vi "split data.vi"(6 "Slide":cluster{dbl, dbl}(slide)={0.0, 1.2121212121212122} scale=-0.00049998..0.0004999999999996373, 7 "dt":dbl, 8 "t0":dbl, 9 "Y(input)":dbl[](array[numeric]), 10 "T(input)":dbl[](array[numeric])) -> (0 "max value":dbl, 1 "min value":dbl, 2 "Y(output)":dbl[](array[numeric]), 3 "T(output)":dbl[](array[numeric]))   [LabVIEW 2014]
panel:
  out "XY Graph":cluster{"T(input)":dbl[], "Y(input) ":dbl[]}(graph)
  out "min index(es)":i32
  out "max index(es)":i32
  out "max":dbl
  out "min":dbl
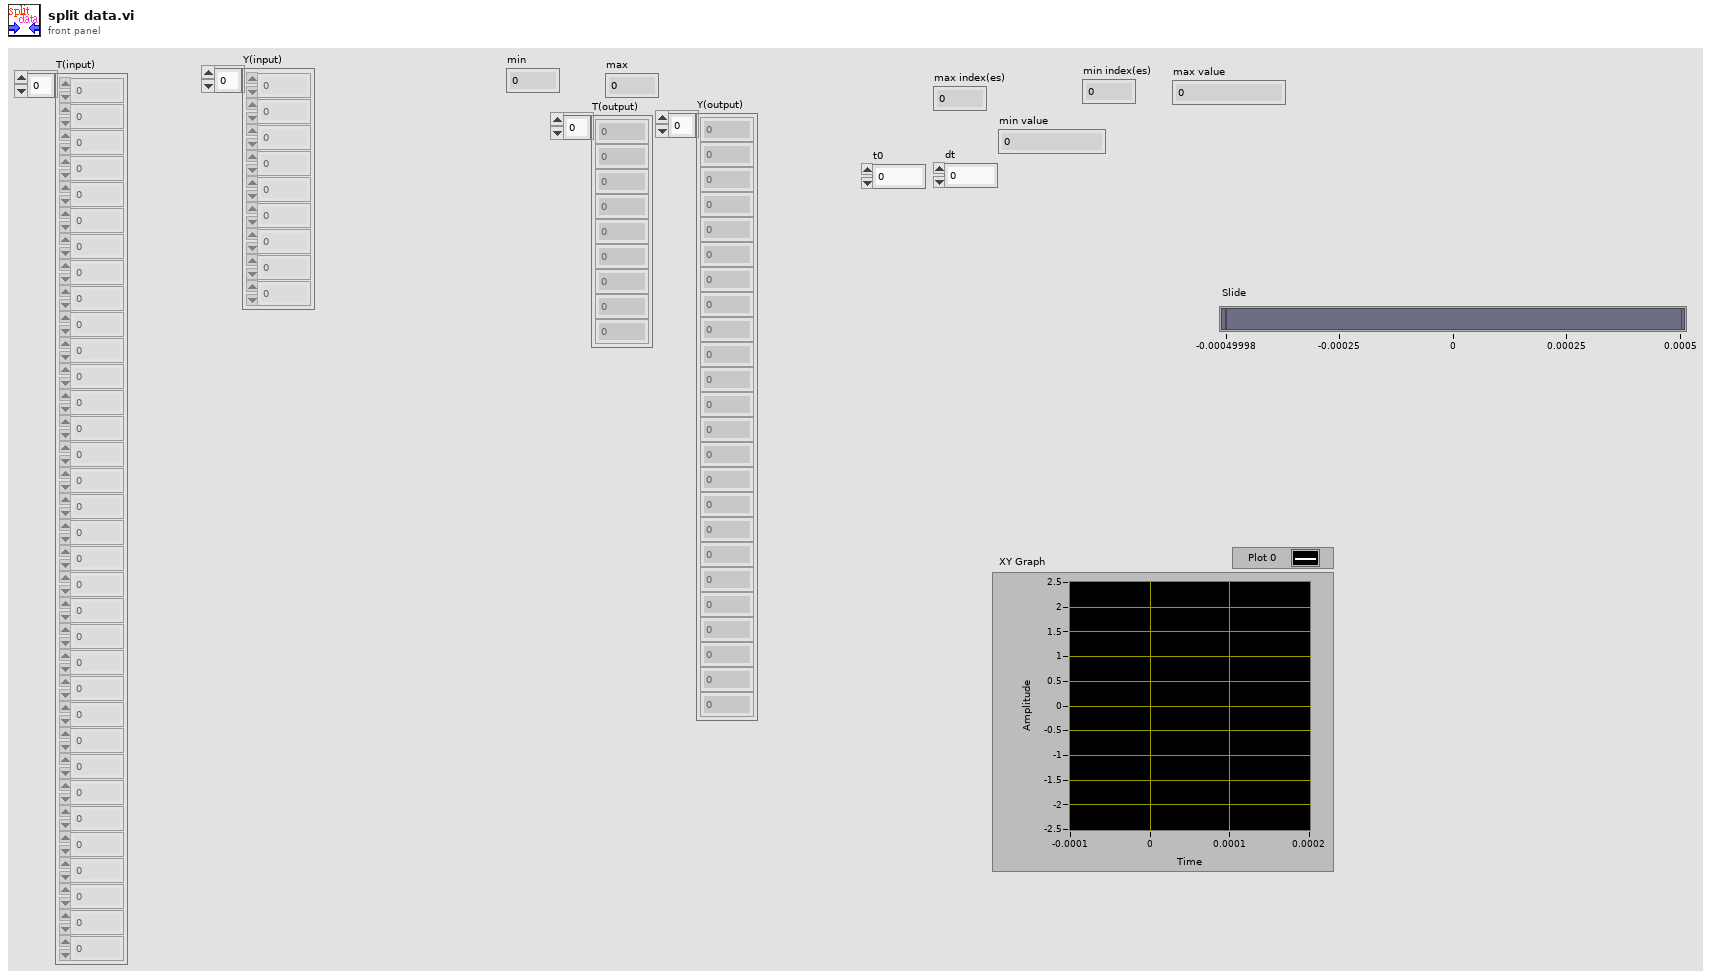
[diagram p1: front panel]
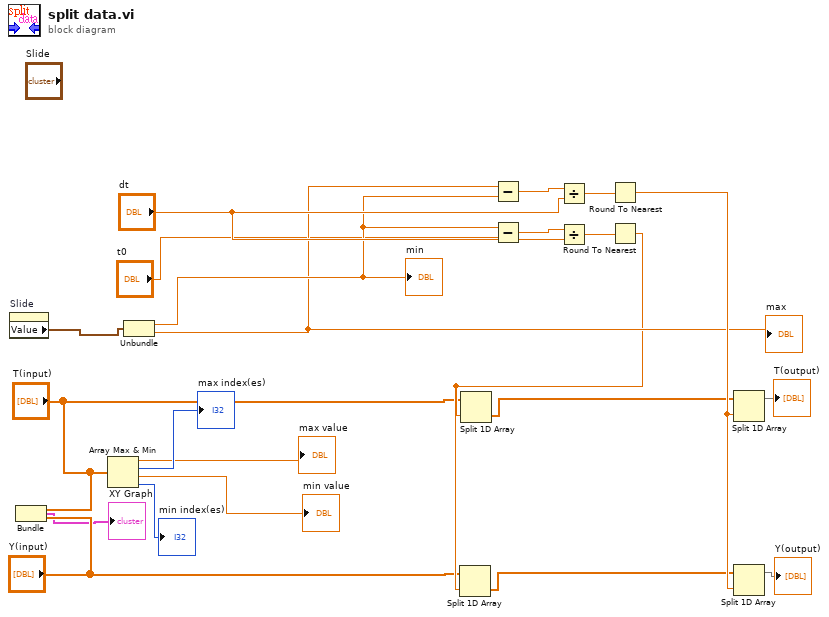
[diagram p0: block diagram]
diagram:
  n1 = property on="Slide" class="Slide (strict)"() -> ("Value"=w6:cluster{dbl, dbl})  [unwired: 2 in, 2 out]
  n2 = Bundle("T(input)"="T(input)", "Y(input)"="Y(input)") -> (→"XY Graph":cluster{"T(input)":dbl[], "Y(input) ":dbl[]})  [unwired: 1 in]
  n3 = Array Max & Min(array="T(input)") -> (max value=→"max value":dbl, max index (indices)=→"max index(es)":i32, min value=→"min value":dbl, min index (indices)=→"min index(es)":i32)
  n4 = Unbundle(w6) -> (w20:dbl, w19:dbl)
  "min" <- w20
  "max" <- w19
  n5 = Subtract(x=w19, y=w20) -> (x-y=w17:dbl)
  n6 = Subtract(x=w20, y="t0") -> (x-y=w14:dbl)
  n7 = Divide(x=w17, y="dt") -> (x/y=w18:dbl)
  n8 = Divide(x=w14, y="dt") -> (x/y=w15:dbl)
  n9 = Round To Nearest(number=w18) -> (nearest integer value=w22:dbl)
  n10 = Round To Nearest(number=w15) -> (nearest integer value=w16:dbl)
  n11 = Split 1D Array(array="Y(input)", index=w16) -> (second subarray=w8:dbl[])  [unwired: 1 out]
  n12 = Split 1D Array(array="T(input)", index=w16) -> (second subarray=w7:dbl[])  [unwired: 1 out]
  n13 = Split 1D Array(array=w7, index=w22) -> (first subarray=→"T(output)":dbl[])  [unwired: 1 out]
  n14 = Split 1D Array(array=w8, index=w22) -> (first subarray=→"Y(output)":dbl[])  [unwired: 1 out]
